vi "Release Notifiers and Queue.vi"(8 "error in":errorcluster, 10 "output cluster":T1) -> (0 "error out":errorcluster)   [LabVIEW 2019, in "DAQmx.lvclass"]
uses:
  DAQmx.lvclass
  typedefs/DAQmx.States--enum.ctl
  typedefs/DAQ.Config.AO--Cluster--Array.ctl
  typedefs/DAQ.Config.AO--Cluster.ctl
  typedefs/DAQ.Config.AO.Range--enum.ctl
  typedefs/DAQ.Config.Device Type--enum.ctl
  typedefs/DAQ.Config.AI--Cluster--Array.ctl
  typedefs/DAQ.Config.AI--Cluster.ctl
  typedefs/DAQ.Config.AI.Coupling--enum.ctl
  typedefs/DAQ.Config.AI.Range--enum.ctl
  typedefs/DAQ.Config.Timing--Cluster.ctl
  typedefs/DAQ.Config.Timing.Sampling--Cluster.ctl
  typedefs/DAQ.Config.Timing.Fs Mode--enum.ctl
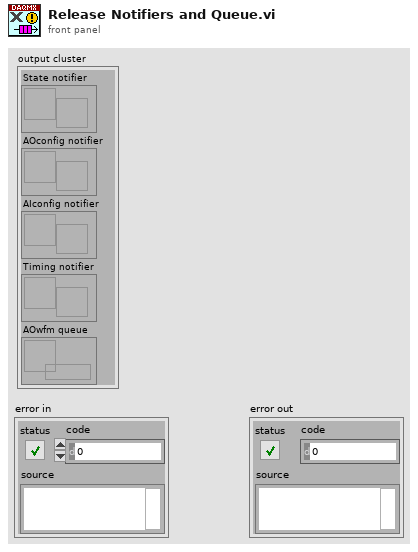
[diagram p1: front panel]
types:
  T1 = cluster{"State notifier":refnum<notifier>, "AOconfig notifier":refnum<notifier>, "AIconfig notifier":refnum<notifier>, "Timing notifier":refnum<notifier>, "AOwfm queue":refnum<queue>}
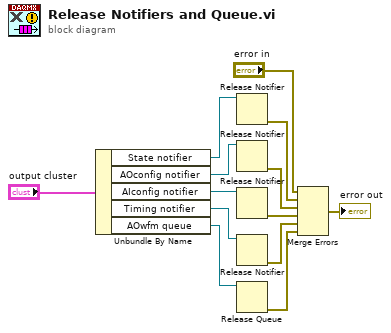
[diagram p0: block diagram]
diagram:
  n1 = Unbundle By Name("output cluster") -> ("State notifier"=w12:refnum<notifier>, "AOconfig notifier"=w11:refnum<notifier>, "AIconfig notifier"=w10:refnum<notifier>, "Timing notifier"=w9:refnum<notifier>, "AOwfm queue"=w8:refnum<queue>)
  n2 = Release Notifier(notifier=w12) -> (error out=w3:errorcluster)  [unwired: 2 in, 2 out]
  n3 = Release Notifier(notifier=w11) -> (error out=w4:errorcluster)  [unwired: 2 in, 2 out]
  n4 = Release Notifier(notifier=w10) -> (error out=w5:errorcluster)  [unwired: 2 in, 2 out]
  n5 = Release Notifier(notifier=w9) -> (error out=w6:errorcluster)  [unwired: 2 in, 2 out]
  n6 = Release Queue(queue=w8) -> (error out=w7:errorcluster)  [unwired: 2 in, 2 out]
  n7 = Merge Errors("error in", w3, w4, w5, w6, w7) -> (→"error out":errorcluster)
